vi "2. Simple State Machine Traffic Light.vi"() -> ()   [LabVIEW 2017]
panel:
  out "millisecond timer value":u32
  in  "stop":bool
  out "Green":bool
  out "Yellow":bool
  out "Red":bool
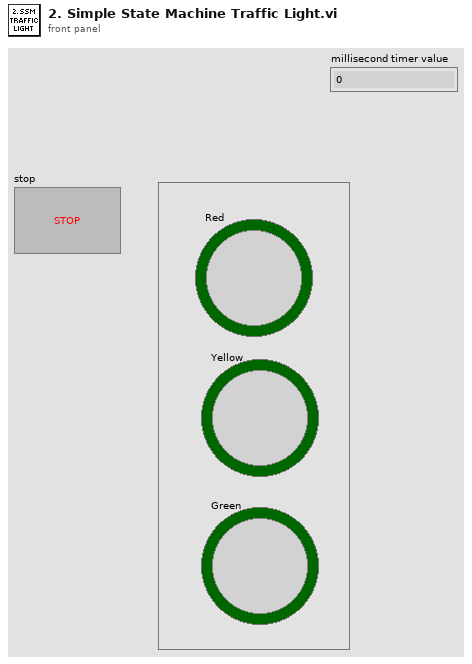
[diagram p1: front panel]
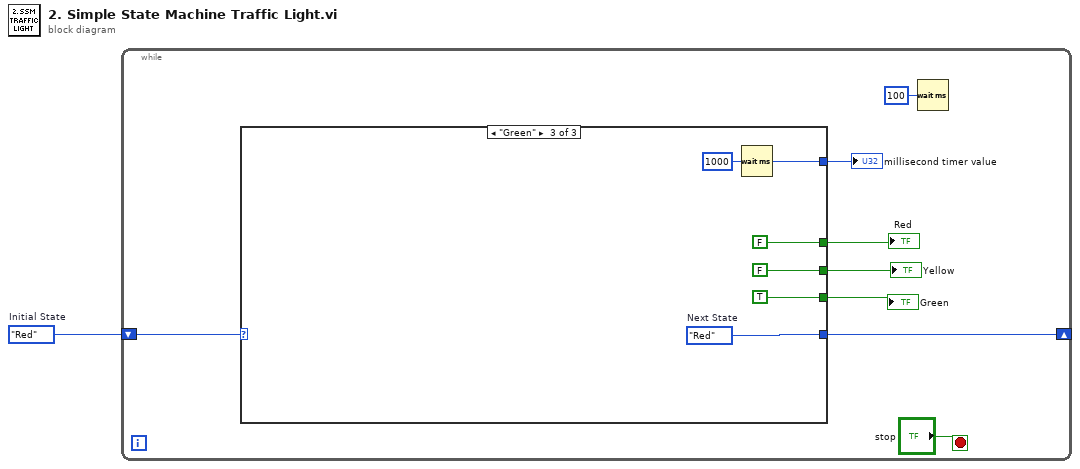
[diagram p0: block diagram]
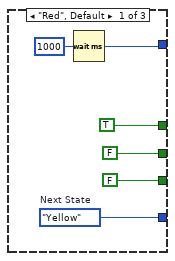
[diagram p2: hidden frame]
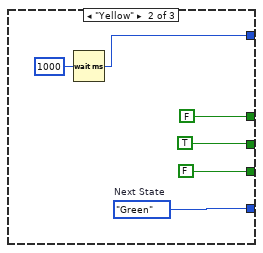
[diagram p3: hidden frame]
diagram:
  w1 = enum16{"Red", "Yellow", "Green"}."Red"  # Initial State
  n1 = while {
    shift-right: [w8] -> _
    shift-left: w1 -> [w9]
    stop <- "stop" stop-if-true
    n2 = case shown="\"Green\"" w9 {
      tunnel: [TRUE FALSE FALSE] -> w3
      tunnel: [w14 w20 w26] -> w8
      tunnel: [FALSE TRUE FALSE] -> w5
      tunnel: [FALSE FALSE TRUE] -> w4
      tunnel: [w10 w16 w22] -> w2
      frame "Red", Default {
        w14 = enum16{"Red", "Yellow", "Green"}."Yellow"  # Next State
        n3 = Wait (ms)(milliseconds to wait=u32 1000) -> (millisecond timer value=w10:u32)
      }
      frame "Yellow" {
        w20 = enum16{"Red", "Yellow", "Green"}."Green"  # Next State
        n4 = Wait (ms)(milliseconds to wait=u32 1000) -> (millisecond timer value=w16:u32)
      }
      frame "Green" {
        w26 = enum16{"Red", "Yellow", "Green"}."Red"  # Next State
        n5 = Wait (ms)(milliseconds to wait=u32 1000) -> (millisecond timer value=w22:u32)
      }
    }
    "Red" <- w3
    "Yellow" <- w5
    "Green" <- w4
    "millisecond timer value" <- w2
    n6 = Wait (ms)(milliseconds to wait=u32 100) -> ()  [unwired: 1 out]
  }
